vi "TI_Debug_Window.vi"() -> ()   [LabVIEW 2011]
uses:
  INA231/Global Variables.vi
panel:
  out "String":string
  in  "Clear":bool
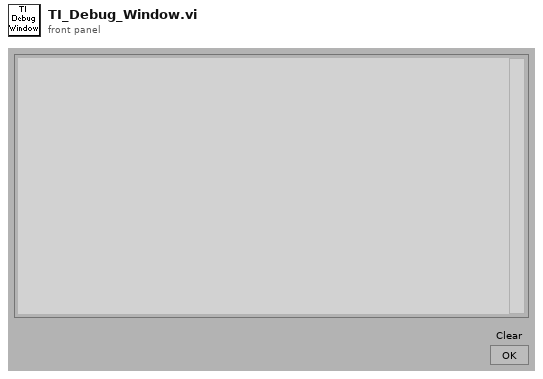
[diagram p1: front panel]
types:
  T1 = enum32{"Invalid", "Standard", "Closed", "Hidden", "Minimized", "Maximized"}
  T2 = enum16{"Always On", "Always Off", "Off While Running"}
  T3 = enum32{"invalid app kind", "Development System", "Run Time System", "Student Edition", "Embedded LabVIEW", "Evaluation", "Custom"}
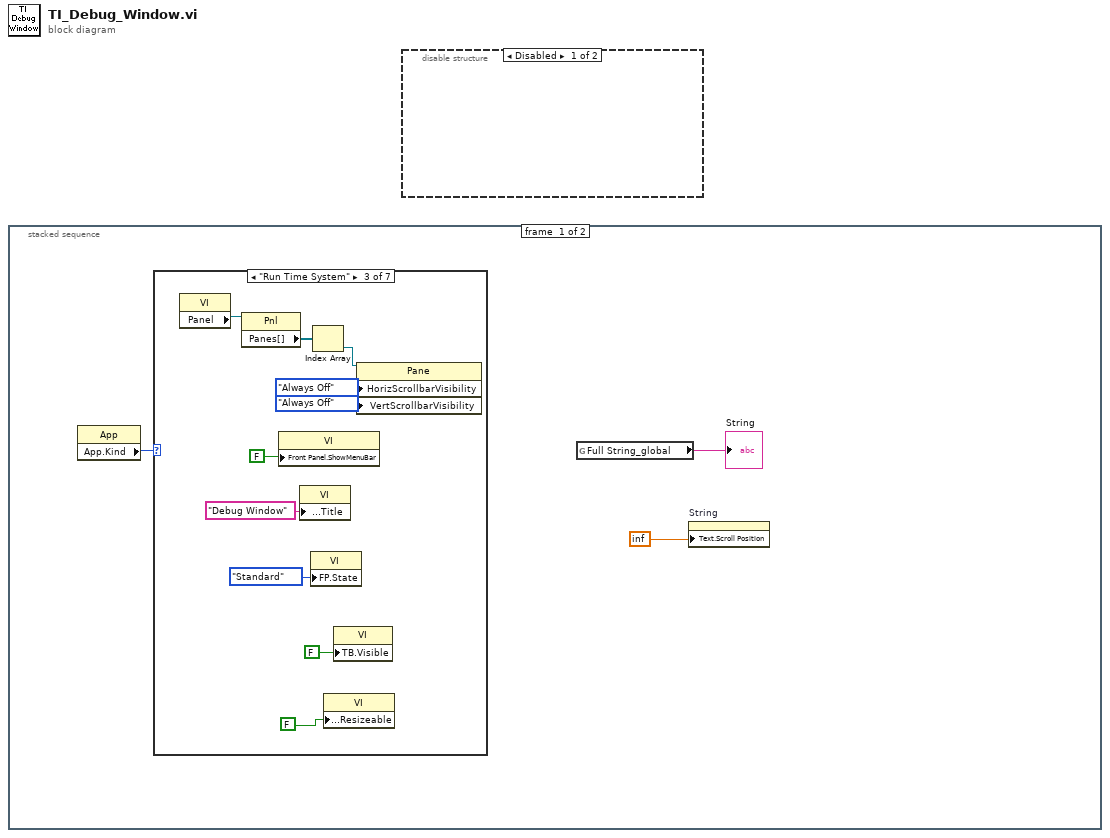
[diagram p0: block diagram]
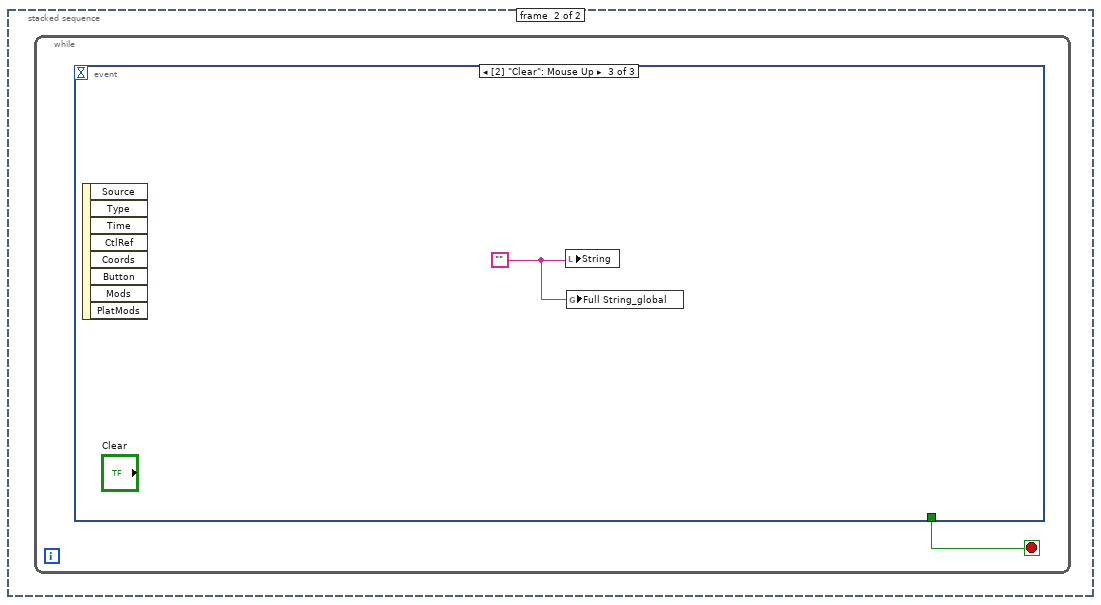
[diagram p9: hidden frame]
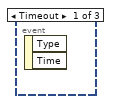
[diagram p10: hidden frame]
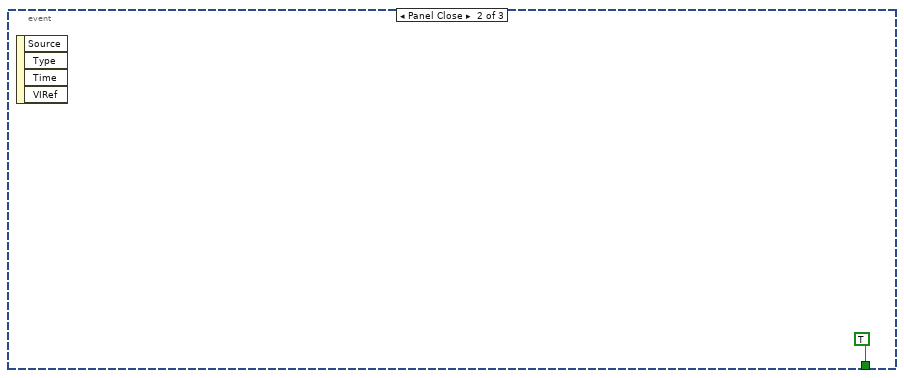
[diagram p11: hidden frame]
diagram:
  n1 = stacked-sequence {
    frame #0 {
      n2 = property class="App"() -> ("App.Kind"=w3:T3)  [unwired: 2 in, 2 out]
      n3 = case shown="\"Run Time System\"" w3 {
        frame "invalid app kind", Default {
        }
        frame "Development System" {
        }
        frame "Run Time System" {
          n4 = property class="VI"() -> ("Panel"=w13:refnum<vi>)  [unwired: 2 in, 2 out]
          n5 = property class="Pnl"(reference=w13) -> ("Panes[]"=w12:refnum<vi>[])  [unwired: 1 in, 2 out]
          n6 = property class="VI"("Front Panel.ShowMenuBar"=FALSE ("Front Panel Window:Show Menu Bar")) -> ()  [unwired: 2 in, 2 out]
          n7 = property class="VI"("Front Panel.Title"="Debug Window" ("Front Panel Window:Title")) -> ()  [unwired: 2 in, 2 out]
          n8 = property class="VI"("FP.State"=T1."Standard" ("Front Panel Window:State")) -> ()  [unwired: 2 in, 2 out]
          n9 = Index Array(array=w12) -> (element=w11:refnum<vi>)  [unwired: 1 in]
          n10 = property class="VI"("Front Panel.Resizeable"=FALSE ("Front Panel Window:Resizeable")) -> ()  [unwired: 2 in, 2 out]
          n11 = property class="VI"("TB.Visible"=FALSE ("Front Panel Window:Resizeable")) -> ()  [unwired: 2 in, 2 out]
          n12 = property class="Pane"(reference=w11, "HorizScrollbarVisibility"=T2."Always Off" ("Horizontal Scrollbar Visibility"), "VertScrollbarVisibility"=T2."Always Off" ("Vertical Scrollbar Visibility")) -> ()  [unwired: 1 in, 2 out]
        }
        frame "Student Edition" {
        }
        frame "Embedded LabVIEW" {
        }
        frame "Evaluation" {
        }
        frame "Custom" {
        }
      }
      n13 = global read "Global Variables.vi" "Full String_global"() -> (→"String":string)
      n14 = property on="String" class="Str"("Text.Scroll Position"=inf) -> ()  [unwired: 2 in, 2 out]
    }
    frame #1 {
      n15 = while {
        stop <- w14 stop-if-true
        n16 = event shown="[2] \"Clear\": Mouse Up" {
          selector: _ -> [_ _ _]
          dyn-events: _ -> [_ _ _]
          timeout: _ -> [_ _ _]
          tunnel: [_ TRUE _] -> w14
          event Timeout {
            n17 = event-data() -> ()  [unwired: 1 in, 2 out]
          }
          event Panel Close {
            n18 = event-data() -> ()  [unwired: 1 in, 4 out]
          }
          event "Clear": Mouse Up {
            w16 = ""
            n19 = event-data() -> ()  [unwired: 1 in, 8 out]
            n20 = local write "String"(w16) -> ()
            n21 = global write "Global Variables.vi" "Full String_global"(w16) -> ()
          }
        }
      }
    }
  }
  n22 = disable-structure shown="Disabled" {
    frame Disabled {
    }
    frame Enabled {
    }
  }
